vi "Set input current_ChSource.vi"(0 "channel name":string, 4 "res(input)":dbl=110.0, 6 "the optimum current(input)":dbl format="%#_6f", 7 "accuracy (input)":dbl step=0.01, 8 "instrument handle":refnum<k15>, 9 "the upper limit for the voltage":dbl=5.0, 10 "Start voltage":dbl=3.0 format="%#.7f", 11 "the lower limit for the voltage":dbl=1.0) -> (1 "current value, mA":dbl, 2 "Error message":string, 3 "the voltage drop across the resistor":dbl=1.1, 5 "accommodated voltage (out)":dbl)   [LabVIEW 2013]
panel:
  out "CH1_Uпит, mA":dbl=15.418111291908591 caption="CH1_AO, ìA" format="%_6g"
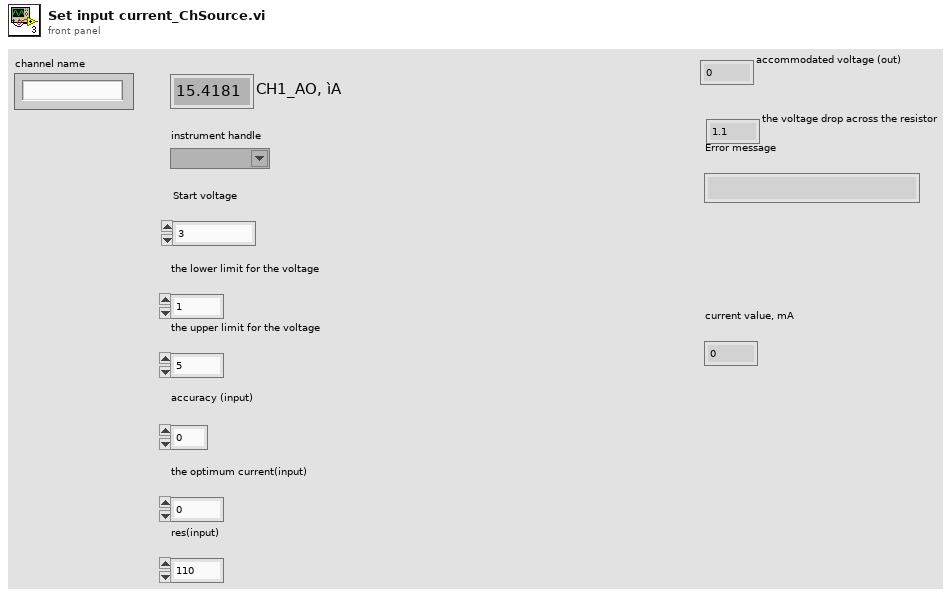
[diagram p1: front panel]
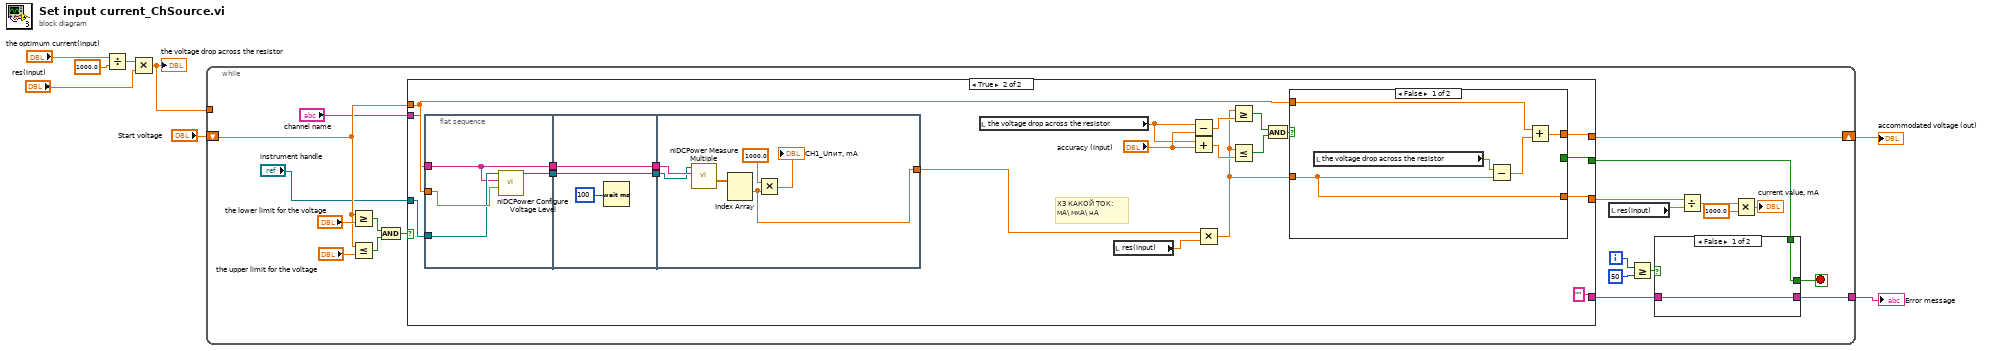
[diagram p0: block diagram]
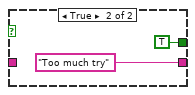
[diagram p2: hidden frame]
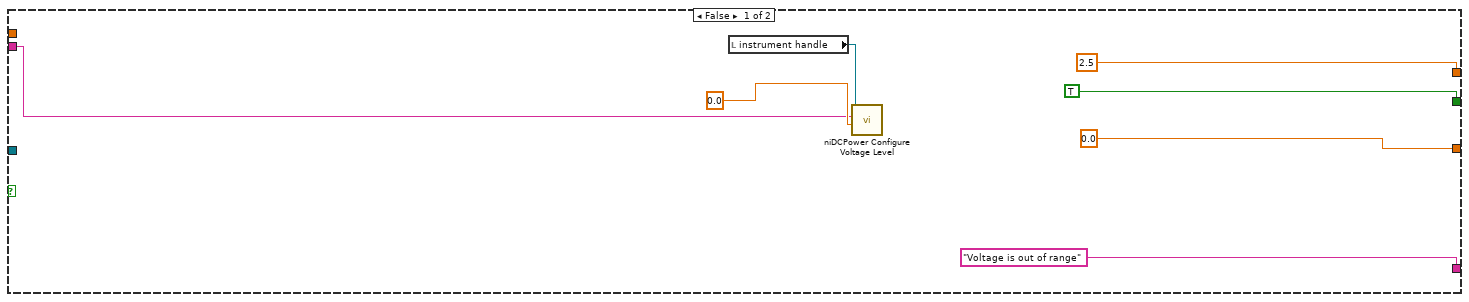
[diagram p3: hidden frame]
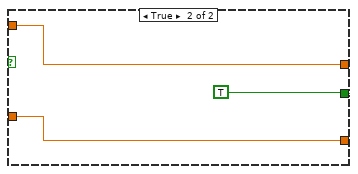
[diagram p4: hidden frame]
diagram:
  n1 = Divide(x="the optimum current(input)", y=1000.0) -> (x/y=w5:dbl)
  n2 = Multiply(x=w5, y="res(input)") -> (x*y=w1:dbl)
  "the voltage drop across the resistor" <- w1
  n3 = while {
    tunnel: [w13] -> w8
    shift-right: [w19] -> w2
    shift-left: "Start voltage" -> [w20]
    tunnel: w1 -> [_]
    i -> [w16]
    stop <- w12 stop-if-true
    n4 = Greater Or Equal?(x=w20, y="the lower limit for the voltage") -> (x >= y?=w28:bool)
    n5 = Less Or Equal?(x=w20, y="the upper limit for the voltage") -> (x <= y?=w29:bool)
    n6 = And(x=w28, y=w29) -> (x .and. y?=w25:bool)
    n7 = case shown="True" w25 {
      tunnel: ["Voltage is out of range" ""] -> w14
      tunnel: [2.5 ("accommodated voltage") w53] -> w19
      tunnel: [TRUE w59] -> w11
      tunnel: [0.0 w54] -> w18
      tunnel: w20 -> [_ w49]
      tunnel: "instrument handle" -> [_ w45]
      tunnel: "channel name" -> [w34 w44]
      frame False {
        n8 = local read "instrument handle"() -> (w36:refnum<k15>)
        n9 = call <instrlib>:"niDCPower Configure Voltage Level.vi"("voltage level"=0.0, "channel name"=w34, "instrument handle"=w36) -> ()  [unwired: 7 in, 2 out]
      }
      frame True {
        # "ХЗ КАКОЙ ТОК:\nмА\\ мкА\\ нА"
        n10 = flat-sequence {
          tunnel: w49 -> [w64]
          tunnel: [w65] -> w50
          tunnel: [w62] -> w46
          tunnel: w45 -> [w63]
          tunnel: w44 -> [w62]
          tunnel: w50 -> [w66]
          tunnel: w46 -> [w67]
          tunnel: [w67] -> w42
          tunnel: [w66] -> w41
          tunnel: [w69] -> w43
          tunnel: w42 -> [w72]
          tunnel: w41 -> [w71]
          frame #0 {
            n11 = call <instrlib>:"niDCPower Configure Voltage Level.vi"("voltage level"=w64, "channel name"=w62, "instrument handle"=w63) -> ("instrument handle out"=w65:refnum<k15>)  [unwired: 7 in, 1 out]
          }
          frame #1 {
            n12 = Wait (ms)(milliseconds to wait=u32 100) -> ()  [unwired: 1 out]
          }
          frame #2 {
            n13 = call <instrlib>:"niDCPower Measure Multiple.vi"("channel name"=w72, "instrument handle"=w71) -> ("current measurements"=w74:dbl[])  [unwired: 6 in, 3 out]
            n14 = Index Array(array=w74) -> (element #1=w69:dbl)  [unwired: 2 in, 1 out]
            n15 = Multiply(x=1000.0 ("y"), y=w69) -> (x*y=→"CH1_Uпит, mA":dbl)
          }
        }
        n16 = local read "the voltage drop across the resistor"() -> (w57:dbl)
        n17 = local read "res(input)"() -> (w48:dbl)
        n18 = Subtract(x=w57, y="accuracy (input)") -> (x-y=w61:dbl)
        n19 = Add(x=w57, y="accuracy (input)") -> (x+y=w60:dbl)
        n20 = Multiply(x=w43, y=w48) -> (x*y=w47:dbl)
        n21 = Greater Or Equal?(x=w47, y=w61) -> (x >= y?=w55:bool)
        n22 = Less Or Equal?(x=w47, y=w60) -> (x <= y?=w56:bool)
        n23 = And(x=w55, y=w56) -> (x .and. y?=w52:bool)
        n24 = case shown="False" w52 {
          tunnel: [_ TRUE] -> w59
          tunnel: [w78 w80] -> w53
          tunnel: w47 -> [w76 w81]
          tunnel: [w76 w81] -> w54
          tunnel: w49 -> [w77 w80]
          frame False {
            n25 = local read "the voltage drop across the resistor"() -> (w75:dbl)
            n26 = Subtract(x=w75, y=w76) -> (x-y=w79:dbl)
            n27 = Add(x=w77, y=w79) -> (x+y=w78:dbl)
          }
          frame True {
          }
        }
      }
    }
    n28 = local read "res(input)"() -> (w24:dbl)
    n29 = Greater Or Equal?(x=w16, y=50) -> (x >= y?=w17:bool)
    n30 = case shown="False" w17 {
      tunnel: w14 -> [w31 _]
      tunnel: [w31 "Too much try"] -> w13
      tunnel: [w30 TRUE] -> w12
      tunnel: w11 -> [w30 _]
      frame False {
      }
      frame True {
      }
    }
    n31 = Divide(x=w18, y=w24) -> (x/y=w23:dbl)
    n32 = Multiply(x=w23, y=1000.0) -> (x*y=→"current value, mA":dbl)
  }
  "Error message" <- w8
  "accommodated voltage (out)" <- w2
